vi "Save Image with ROI Data.vi"() -> ()   [LabVIEW 2009]
panel:
  out "Image 2":T1(plugin-control)
  in  "source":path
  out "Image":T1(plugin-control)
  in  "Destination Path":path
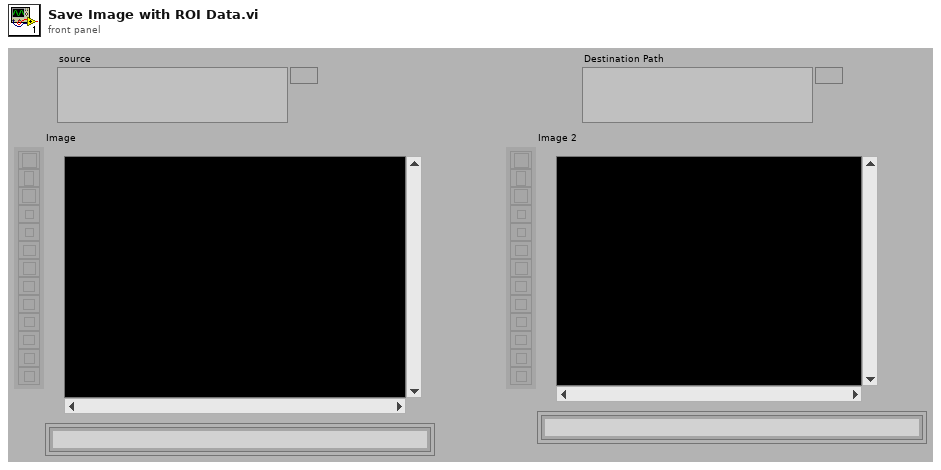
[diagram p1: front panel]
types:
  T1 = typedef "IMAQ Image.ctl" = refnum<image>
  T2 = typedef "ROI Descriptor" = cluster{"Global Rectangle":i32[], "Contours":cluster{"ID":enum32{"External", "Internal"}, "Type":u32, "Coordinates":i32[]}[]}
  T3 = typedef "IMAQ Rectangle" = cluster{"Left":i32, "Top":i32, "Right":i32, "Bottom":i32, "Rotation":dbl}
  T4 = cluster{"Left":i32, "Top":i32, "Right":i32, "Bottom":i32}
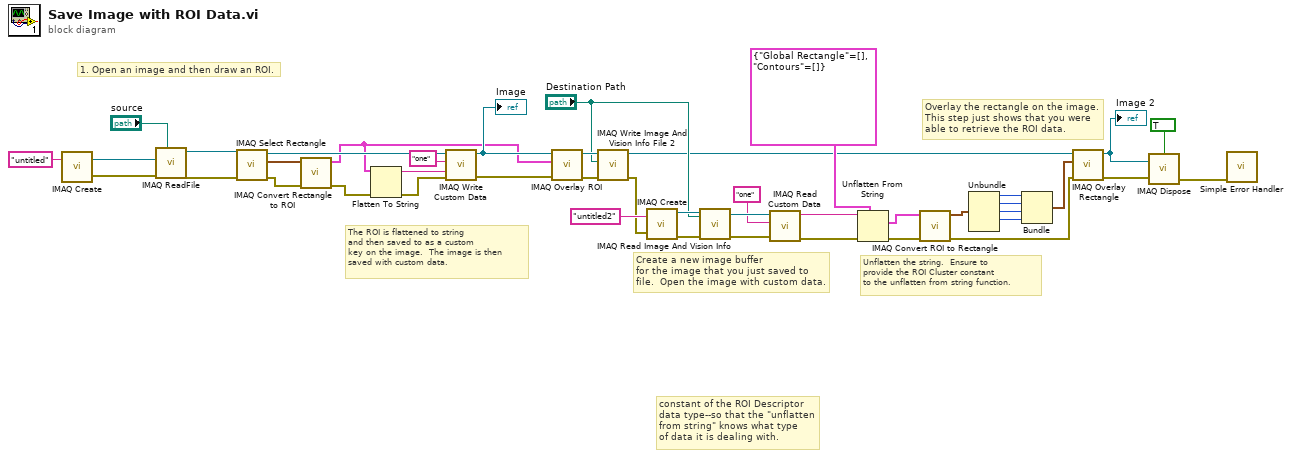
[diagram p0: block diagram]
diagram:
  # "Overlay the rectangle on the image. \nThis step just shows that you were \nable to retrieve the ROI data."
  # "Unflatten the string.  Ensure to\nprovide the ROI Cluster constant \nto the unflatten from string function."
  # "Create a new image buffer\nfor the image that you just saved to\nfile.  Open the image with custom data."
  # "The ROI is flattened to string \nand then saved to as a custom\nkey on the image.  The image is then \nsaved with custom data."
  # "1. Open an image and then draw an ROI."
  # "constant of the ROI Descriptor\ndata type--so that the \"unflatten\nfrom string\" knows what type \nof data it is dealing with."
  n1 = call "IMAQ Create"("Image Name"="untitled") -> ("New Image"=w43:T1, "error out"=w42:errorcluster)  [unwired: 4 in]
  n2 = call "IMAQ ReadFile"("File Path"="source", "error in (no error)"=w42, "Image"=w43) -> ("error out"=w39:errorcluster, "Image Out"=w40:T1)  [unwired: 4 in, 3 out]
  n3 = call "IMAQ Select Rectangle"("error in (no error)"=w39, "Image In"=w40) -> ("error out"=w37:errorcluster, "Rectangle"=w38:T3, "Image Out (duplicate)"=w31:T1)  [unwired: 6 in, 1 out]
  n4 = call "IMAQ Convert Rectangle to ROI"("error in (no error)"=w37, "Rectangle"=w38) -> ("error out"=w28:errorcluster, "ROI Descriptor"=w16:T2)  [unwired: 7 in]
  n5 = Flatten To String(anything=w16, error in (no error)=w28) -> (data string=w23:string, error out=w29:errorcluster)  [unwired: 2 in, 1 out]
  n6 = call "IMAQ Write Custom Data"("error in (no error)"=w29, "Custom Data In"=w23, "Key"="one", "Image"=w31) -> ("error out"=w27:errorcluster, "Image Out"=w26:T1)  [unwired: 6 in]
  "Image" <- w26
  n7 = call "IMAQ Overlay ROI"("error in (no error)"=w27, "ROI Descriptor"=w16, "Image"=w26) -> ("error out"=w35:errorcluster, "Image Out"=w32:T1)  [unwired: 7 in]
  n8 = call "IMAQ Write Image And Vision Info File 2"("error in (no error)"=w35, "File Path"="Destination Path", "Image"=w32) -> ("error out"=w14:errorcluster, "Image Out (duplicate)"=w2:T1)  [unwired: 7 in]
  n9 = call "IMAQ Create"("Image Name"="untitled2", "error in (no error)"=w14) -> ("New Image"=w25:T1, "error out"=w13:errorcluster)  [unwired: 3 in]
  n10 = call "IMAQ Read Image And Vision Info"("File Path"="Destination Path", "error in (no error)"=w13, "Image"=w25) -> ("error out"=w21:errorcluster, "Image Out"=w22:T1)  [unwired: 6 in, 1 out]
  n11 = call "IMAQ Read Custom Data"("error in (no error)"=w21, "Key"="one", "Image"=w22) -> ("error out"=w17:errorcluster, "Custom Data Out"=w19:string)  [unwired: 6 in, 1 out]
  n12 = Unflatten From String(type=T2 {"Global Rectangle"=[], "Contours"=[]} ("ROI Descriptor"), binary string=w19, error in (no error)=w17) -> (value=w11:T2, error out=w12:errorcluster)  [unwired: 2 in, 1 out]
  n13 = call "IMAQ Convert ROI to Rectangle"("error in (no error)"=w12, "ROI Descriptor"=w11) -> ("error out"=w1:errorcluster, "Rectangle"=w10:T3)  [unwired: 7 in]
  n14 = Unbundle(w10) -> ("Left"=w9:i32, "Top"=w8:i32, "Right"=w7:i32, "Bottom"=w6:i32)  [unwired: 1 out]
  n15 = Bundle("Left"=w9, "Top"=w8, "Right"=w7, "Bottom"=w6) -> (w5:T4)  [unwired: 1 in]
  n16 = call "IMAQ Overlay Rectangle"("error in (no error)"=w1, "Rectangle"=w5, "Image"=w2) -> ("error out"=w4:errorcluster, "Image Out"=w3:T1)  [unwired: 7 in]
  "Image 2" <- w3
  n17 = call "IMAQ Dispose"("All Images? (No)"=TRUE, "Image"=w3, "error in (no error)"=w4) -> ("error out"=w15:errorcluster)  [unwired: 3 in]
  n18 = call <vilib>:"Simple Error Handler.vi"("error in (no error)"=w15) -> ()  [unwired: 4 in, 5 out]
